vi "processing.vi"(4 "Kernel div":dbl, 6 "Color channel":T1, 7 "Kernel":dbl[][](array[numeric]), 9 "Columns":i32, 10 "Rows":i32, 11 "Div":dbl) -> (3 "Result":T1)   [LabVIEW 2016]
uses:
  <vilib>/Analysis/Matrix/Datatypes/RealMatrix.ctl
  <vilib>/Analysis/Matrix/Numeric/Conversions/Matrix To Array - RM.vi
  <vilib>/Analysis/Matrix/NI_Matrix.lvlib
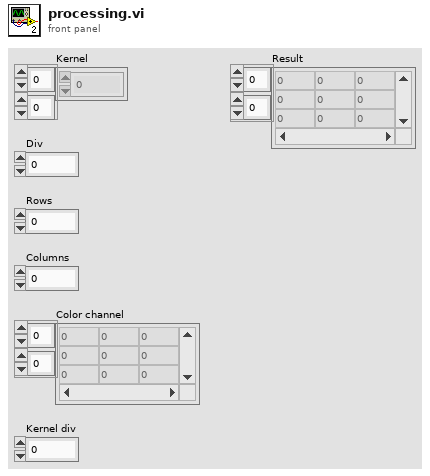
[diagram p1: front panel]
types:
  T1 = typedef "NI_Matrix.lvlib/RealMatrix.ctl" = dbl[][]
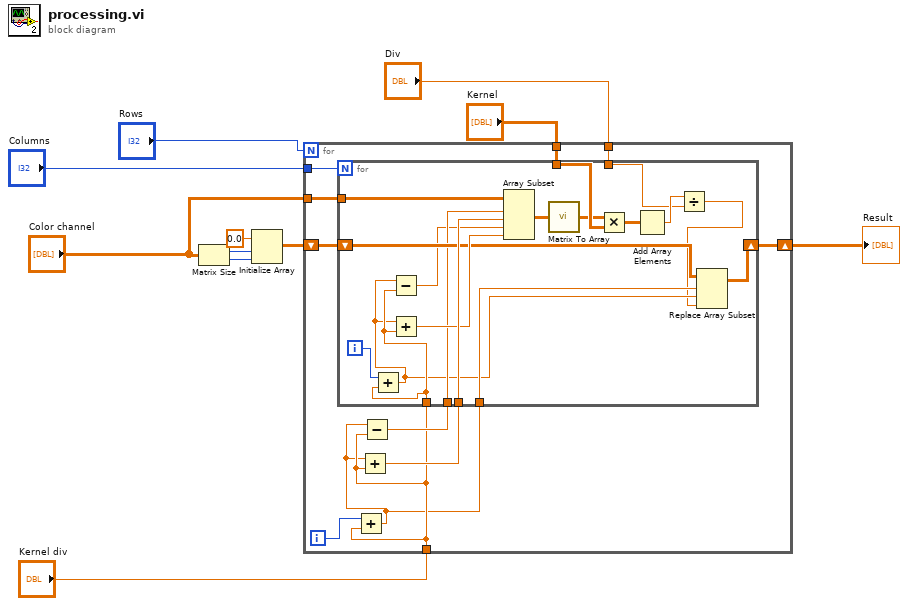
[diagram p0: block diagram]
diagram:
  n1 = Matrix Size(0:"Color channel") -> (1:w2:i32, 2:w3:i32)
  n2 = Initialize Array(0.0 ("element"), w2, w3) -> (w6:dbl[][])
  n3 = for {
    N: "Rows" -> [_]
    tunnel: "Kernel div" -> [w15]
    tunnel: "Kernel" -> [w20]
    tunnel: "Div" -> [w19]
    tunnel: "Color channel" -> [w21]
    shift-right: [w17] -> w7
    shift-left: w6 -> [w18]
    tunnel: "Columns" -> [w12]
    i -> [w14]
    n4 = Add(x=w14, y=w15) -> (x+y=w13:dbl)
    n5 = Add(x=w13, y=w15) -> (x+y=w22:dbl)
    n6 = Subtract(x=w13, y=w15) -> (x-y=w16:dbl)
    n7 = for {
      N: w12 -> [_]
      tunnel: w15 -> [w31]
      tunnel: w16 -> [w34]
      tunnel: w22 -> [w40]
      tunnel: w20 -> [w37]
      tunnel: w19 -> [w26]
      tunnel: w21 -> [w38]
      shift-right: [w35] -> w17
      shift-left: w18 -> [w36]
      tunnel: w13 -> [w30]
      i -> [w32]
      n8 = Add(x=w32, y=w31) -> (x+y=w29:dbl)
      n9 = Subtract(x=w29, y=w31) -> (x-y=w33:dbl)
      n10 = Add(x=w29, y=w31) -> (x+y=w39:dbl)
      n11 = Array Subset(array=w38, index (row)=w34, length (row)=w40, index (col)=w33, length (col)=w39) -> (w24:T1)
      n12 = call-poly <vilib>:"Matrix To Array.vi"("Real Matrix"=w24) -> ("Real 2D Array"=w23:dbl[][])
      n13 = Multiply ("Multiply.vi")(x=w23, y=w37) -> (x*y=w28:dbl[][])
      n14 = Add Array Elements(numeric array=w28) -> (sum=w27:dbl)
      n15 = Divide(x=w27, y=w26) -> (x/y=w25:dbl)
      n16 = Replace Array Subset(array=w36, new element=w25, index (row)=w30, index (col)=w29) -> (w35:T1)
    }
  }
  "Result" <- w7
